vi "Grab Snapshots.vi"() -> ()   [LabVIEW 2019]
doc: "Grab any video source supported by QuickTime (internal, USB, FW, etc).\nThe output image can be compressed with any QT supported format (See image->compressed_data).\nSet Dialogs to 1 in Frame grabber settings to use the standard QT dialog.\n\nChris Salzmann © 1994-2003"
uses:
  Sub VIs/QTLIB_2595.llb/QT_FrameGrabber.ctl
  Sub VIs/QTLIB_2595.llb/QT_Video.ctl
  Sub VIs/QTLIB_2595.llb/QT_Image.ctl
  Sub VIs/QTLIB_2595.llb/QT_Private.ctl
  Sub VIs/QTLIB_2595.llb/QT_File.ctl
  Sub VIs/QTLIB_2595.llb/QT_Compression.ctl
panel:
  in  "Case Constant\n(See Context Help)":bool=TRUE
  in  "File Prefix":string="SnapShot "
  in  "Path":path=path "/Data2Mac/Users/user/Pictures/132_2"
  in  "Snap Shot Timing":dbl[unit]=10.0
  in  "White l.":dbl(slide)=80.61224489795919 scale=0.0..100.0
  in  "Black l.":dbl(slide)=14.285714285714286 scale=0.0..100.0
  in  "Sharp":dbl(slide)=1.7857142857142858 scale=0.0..100.0
  in  "Contr":dbl(slide)=53.57142857142858 scale=0.0..100.0
  in  "Bright":dbl(slide)=53.06122448979592 scale=0.0..100.0
  in  "Sat":dbl(slide)=51.02040816326531 scale=0.0..100.0
  in  "Hue":dbl(slide)=50.0 scale=0.0..100.0
  out "CIN info":string="© Chris 94-2002, QT Fat-CIN, rev: 2576, FATQTCin.c, Jul 11 2003, 14:22:30"
  out "QT Version":string="QuickTime v. 630 "
  in  "stop":bool
  in  "Frame Grabber Settings":T1={"Name"="Tester", "Digitizer"=1, "Input"=1, "Witdh"=768, "Height"=576, "Input format"=enum."NTSC", "Frame rate"=20.0, "Reserved"=0, "Dialogs"=1} {"Frame rate" format="%#1_6g"; "Dialogs" format="%.0b"}
  out "Picture":picture
  # "Grab any video source supported by QuickTime (internal, USB, FW, etc).\nThe output image can be compressed with any QT supported format (See image->compressed_data).\nSet Dialogs to 1 in Frame grabber settings to use the standard QT dialog.\n\nChris Salzmann © 1994-2003"
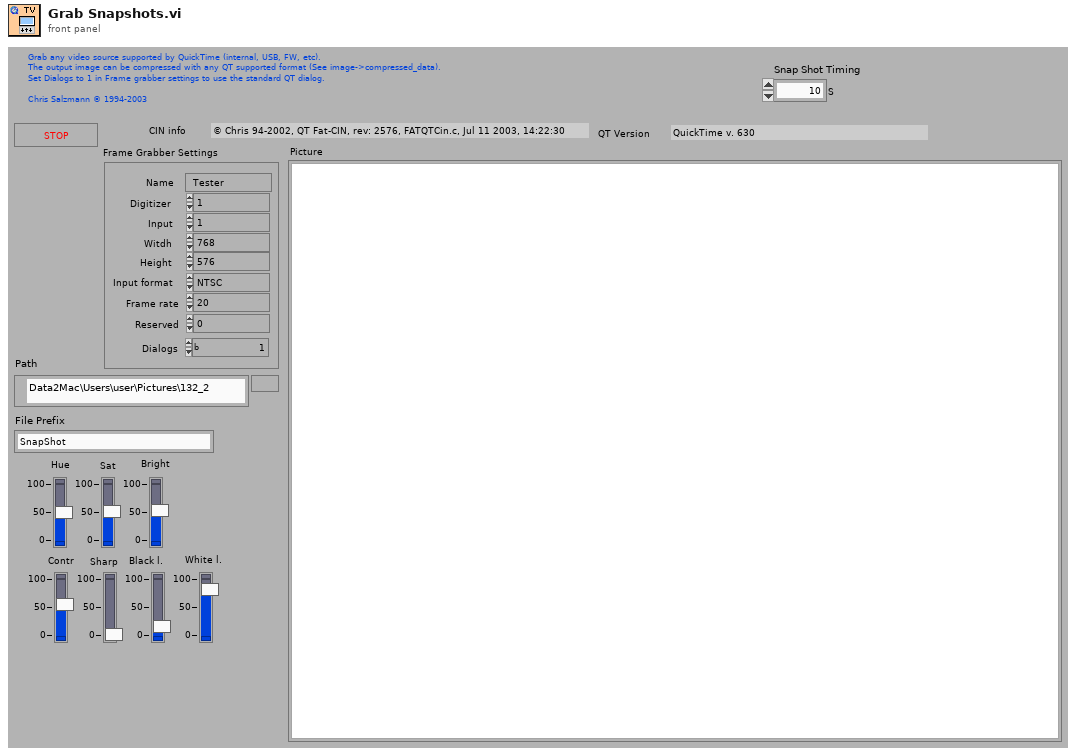
[diagram p1: front panel]
types:
  T1 = typedef "QT_FrameGrabber.ctl" = cluster{"Name":string, "Digitizer":i32, "Input":i32, "Witdh":i32, "Height":i32, "Input format":enum32{"NTSC", "PAL", "Secam"}, "Frame rate":dbl, "Reserved":i32, "Dialogs":u32}
  T2 = typedef "QT_Image.ctl" = cluster{"Witdh":i32, "Height":i32, "Depth":i32, "data":u8[], "Compressed data":u8[], "Color table":u32[], "Duration":i32, "Options":i32, "Timestamp":i32, "ID":i32, "Reserved":i32, "Dialogs":u32}
  T3 = typedef "QT_Compression.ctl" = cluster{"Compression":i32, "Format":i32, "Codec":i32, "Comp. Quality":i32, "Key Frame":i32, "Dialogs":u32}
  T4 = typedef "QT_Video.ctl" = cluster{"Color format":u32, "Hue":dbl, "Saturation":dbl, "Brightness":dbl, "Contrast":dbl, "Sharpness":dbl, "Black Level":dbl, "White Level":dbl, "Options":i32, "Dialogs":u32}
  T5 = typedef "QT_Private.ctl" = cluster{"reserved 1":i32, "reserved 2":i32, "reserved 3":i32, "reserved 4":i32}
  T6 = typedef "QT_File.ctl" = cluster{"Paths":string[], "Options":i32, "Dialogs":u32, "Reserved":i32}
  T7 = typedef "QT_Ref.ctl" = refnum<k1>
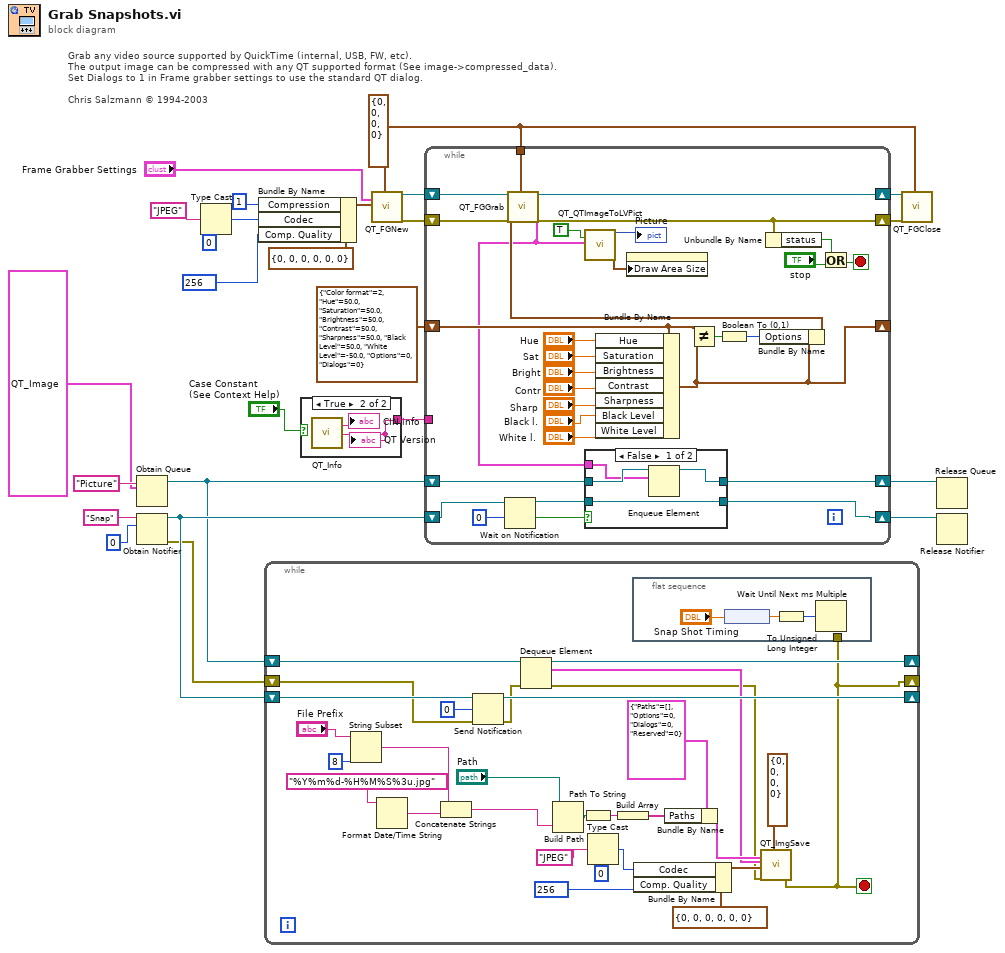
[diagram p0: block diagram]
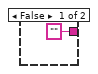
[diagram p3: hidden frame]
diagram:
  w18 = T5 {"reserved 1"=0, "reserved 2"=0, "reserved 3"=0, "reserved 4"=0} ("Private")
  # "Grab any video source supported by QuickTime (internal, USB, FW, etc).\nThe output image can be compressed with any QT supported format (See image->compressed_data).\nSet Dialogs to 1 in Frame grabber settings to use the standard QT dialog.\n\nChris Salzmann © 1994-2003"
  n1 = Obtain Queue(name (unnamed)="Picture", element data type=T2 {"Witdh"=320, "Height"=240, "Depth"=32, "data"=array[307200 elements], "Compressed data"=array[6546 elements], "Color table"=[], "Duration"=0, "Options"=0, "Timestamp"=0, "ID"=525, "Reserved"=0, "Dialogs"=0} ("Image/Movie Out")) -> (queue out=w10:refnum<queue>)  [unwired: 3 in, 2 out]
  n2 = Obtain Notifier(name (unnamed)="Snap", notification data type=0) -> (notifier out=w13:refnum<notifier>, error out=w1:errorcluster)  [unwired: 2 in, 1 out]
  n3 = Type Cast(type=0 ("Format"), x="JPEG") -> (*(type *) &x=w6:i32)
  n4 = Bundle By Name(cluster=T3 {"Compression"=0, "Format"=0, "Codec"=0, "Comp. Quality"=0, "Key Frame"=0, "Dialogs"=0} ("Compression Settings"), "Compression"=1, "Codec"=w6, "Comp. Quality"=256) -> (w20:T3)
  n5 = while {
    shift-right: [w53] -> _
    shift-left: w13 -> [w54]
    shift-right: [w50] -> _
    shift-left: w10 -> [w51]
    shift-right: [w26] -> _
    shift-left: w1 -> [w30]
    stop <- w26 stop-if-true
    n6 = String Subset(string="File Prefix", length (rest)=8 ("length (rest)")) -> (substring=w29:string)  [unwired: 1 in]
    n7 = Format Date/Time String(time format string (%c)="%Y%m%d-%H%M%S%3u.jpg") -> (date/time string=w34:string)  [unwired: 2 in]
    n8 = Concatenate Strings(w29, w34) -> (w32:string)
    n9 = Send Notification(notification=0, notifier=w54, error in (no error)=w30) -> (notifier out=w53:refnum<notifier>, error out=w52:errorcluster)
    n10 = Dequeue Element(queue=w51, error in (no error)=w52) -> (queue out=w50:refnum<queue>, element=w39:T2, error out=w27:errorcluster)  [unwired: 1 in, 1 out]
    n11 = Build Path(base path="Path", name or relative path=w32) -> (appended path=w37:path)
    n12 = Path To String(path=w37) -> (string=w42:string)
    n13 = Type Cast(type=0 ("Format"), x="JPEG") -> (*(type *) &x=w48:i32)
    n14 = Build Array(w42) -> (w49:string[])
    n15 = flat-sequence {
      tunnel: w26 -> [_]
      frame #0 {
        n16 = node("Snap Shot Timing") -> (w56:dbl)
        n17 = To Unsigned Long Integer(number=w56) -> (unsigned 32bit integer=w55:u32)
        n18 = Wait Until Next ms Multiple(millisecond multiple=w55) -> ()  [unwired: 1 out]
      }
    }
    n19 = Bundle By Name(cluster=T3 {"Compression"=0, "Format"=0, "Codec"=0, "Comp. Quality"=0, "Key Frame"=0, "Dialogs"=0} ("Compression Settings"), "Codec"=w48, "Comp. Quality"=256) -> (w44:T3)
    n20 = Bundle By Name(cluster=T6 {"Paths"=[], "Options"=0, "Dialogs"=0, "Reserved"=0} ("File Settings"), "Paths"=w49) -> (w46:T6)
    n21 = call "QT_ImgSave.vi"("File Settings"=w46, "Image In"=w39, "Compression Settings"=w44, "error in (no error)"=w27, "Private"=T5 {"reserved 1"=0, "reserved 2"=0, "reserved 3"=0, "reserved 4"=0}) -> ("error out"=w26:errorcluster)  [unwired: 14 in]
  }
  n22 = case shown="True" "Case Constant\n(See Context Help)" {
    tunnel: ["" ("QT Version") w60] -> w17
    frame False {
    }
    frame True {
      n23 = call "QT_Info.vi"() -> ("CIN info"=→"CIN info":string, "QT Version"=w60:string)  [unwired: 13 in, 5 out]
      "QT Version" <- w60
    }
  }
  n24 = call "QT_FGNew.vi"("Frame Grabber Settings"="Frame Grabber Settings", "Compression Settings"=w20, "Private"=w18) -> ("QT Ref Out"=w25:T7, "error out"=w21:errorcluster)  [unwired: 15 in]
  n25 = while {
    shift-left: T4 {"Color format"=2, "Hue"=50.0, "Saturation"=50.0, "Brightness"=50.0, "Contrast"=50.0, "Sharpness"=50.0, "Black Level"=50.0, "White Level"=-50.0, "Options"=0, "Dialogs"=0} ("Video Settings") -> [w78]
    shift-right: [w76] -> _
    tunnel: w18 -> [w90]
    tunnel: w17 -> [_]
    shift-right: [w66] -> w3
    shift-left: w13 -> [w70]
    shift-right: [w65] -> w2
    shift-left: w10 -> [w64]
    shift-right: [w61] -> w12
    shift-left: w21 -> [w89]
    shift-right: [w62] -> w11
    shift-left: w25 -> [w91]
    stop <- w88 stop-if-true
    n26 = Wait on Notification(notifier=w70, timeout in ms (-1)=0) -> (notifier out=w67:refnum<notifier>, timed out?=w68:bool)  [unwired: 2 in, 2 out]
    n27 = Bundle By Name(cluster=w78, "Hue"="Hue", "Saturation"="Sat", "Brightness"="Bright", "Contrast"="Contr", "Sharpness"="Sharp", "Black Level"="Black l.", "White Level"="White l.") -> (w76:T4)
    n28 = Not Equal?(x=w78, y=w76) -> (x != y?=w77:bool)
    n29 = Boolean To (0,1)(Boolean=w77) -> (0, 1=w71:i16)
    n30 = Bundle By Name(cluster=w76, "Options"=w71) -> (w75:T4)
    n31 = call "QT_FGGrab.vi"("QT Ref In"=w91, "Video Settings in"=w75, "error in (no error)"=w89, "Private"=w90) -> ("QT Ref Out"=w62:T7, "Image/Movie Out"=w63:T2, "error out"=w61:errorcluster)  [unwired: 12 in, 1 out]
    n32 = call "QT_QTImageToLVPict.vi"("Draw info"=TRUE, "Image/Movie Out"=w63) -> ("Picture color"=→"Picture":picture, "Pict Draw Area Size"=w72:cluster{"Width":i16, "Height":i16})  [unwired: 13 in, 3 out]
    n33 = case shown="False" w68 {
      tunnel: w67 -> [w95 w97]
      tunnel: [w95 w97] -> w66
      tunnel: w64 -> [w93 w96]
      tunnel: [w94 w96] -> w65
      tunnel: w63 -> [w92 _]
      frame False {
        n34 = Enqueue Element(queue=w93, element=w92) -> (queue out=w94:refnum<queue>)  [unwired: 2 in, 2 out]
      }
      frame True {
      }
    }
    n35 = property on="Picture" class="Pict"("Draw Area Size"=w72) -> ()  [unwired: 2 in, 2 out]
    n36 = Unbundle By Name(w61) -> ("status"=w86:bool)
    n37 = Or(x=w86, y="stop") -> (x .or. y?=w88:bool)
  }
  n38 = call "QT_FGClose.vi"("QT Ref In"=w11, "error in (no error)"=w12, "Private"=w18) -> ()  [unwired: 15 in, 2 out]
  n39 = Release Queue(queue=w2) -> ()  [unwired: 2 in, 3 out]
  n40 = Release Notifier(notifier=w3) -> ()  [unwired: 2 in, 3 out]
